vi "Simple SFTP File Download.vi"() -> ()   [LabVIEW 2018]
doc: "Downloads, or receives, a relatively small file from a remote SFTP server. This is similar to the SFTP command line utility when transferring, or copying, a remote file to a local destination. If performance is poor or memory is limited on the local machine, then it could be because the file is relatively large and this implementation is not very efficient for relatively large files."
uses:
  Toolkit/SFTP Attributes/SFTP Attributes.lvclass/SFTP Attributes.ctl
  Toolkit/SSH/SSH.lvclass/SSH.ctl
  Toolkit/SSH/Utility/Read Shared Library.vi
  Toolkit/Session/Support/Create from SSH.vi
  Toolkit/Session/Support/Password Authentication.vi
  Toolkit/SFTP/Support/Create from Session.vi
  Toolkit/SFTP File/Support/Open from SFTP.vi
  Toolkit/SFTP Attributes/Support/Create from SFTP File.vi
  Toolkit/Support/Check Status.vi
  Toolkit/SFTP Attributes/Support/Destroy to SFTP File.vi
  Toolkit/SFTP File/Support/Close to SFTP.vi
  Toolkit/SFTP/Support/Destroy to Session.vi
  Toolkit/Session/Support/Destroy to SSH.vi
  Toolkit/SSH/SSH.lvclass
  Toolkit/Session/Session.lvclass
  Toolkit/SFTP/SFTP.lvclass
  Toolkit/SFTP File/SFTP File.lvclass
  Toolkit/SFTP Attributes/SFTP Attributes.lvclass
panel:
  in  "Remote File":string
  in  "Local File":path
  in  "Remote SFTP Server":string
  in  "Password":string
  in  "Username":string
  # "Overview: Demonstrates transferring, or downloading, a remote file from a SSH server, similar to the SFTP command line utility\nInstructions:\n1. Enter the IP address or host name of the remote SFTP server. This can be a CompactRIO (cRIO) running the National Instruments Linux Real-Time (NI Linux RT) operating system with the Enable Secure Shell Server (sshd) checkbox checked. \n2. Enter a username. If using a cRIO with a default configuration, then the username is \"admin\".\n3. Enter a password for the username. If using a cRIO with a default configuration, then the password is blank (empty).\n4. Enter the path and/or filename of the remote file to download. Typically, this is a POSIX/UNIX file path with a backslash, \"/\", used to separate directories and the default directory is the remote user's home directory, i.e. \"/home/admin\" on a default configured cRIO.\n5. Select a destination on the local computer for the transfer/download from the remote SSH server.\n6. Run this VI."
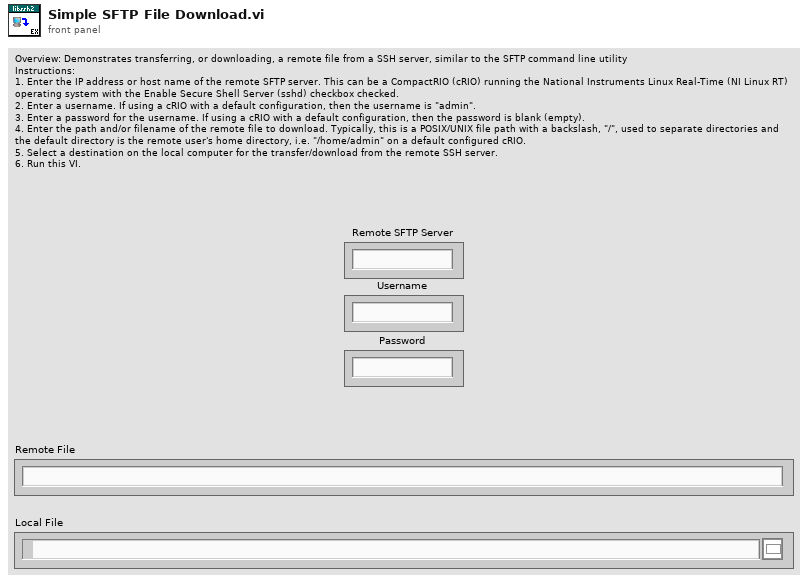
[diagram p1: front panel]
types:
  T1 = enum16{"open", "replace", "create", "open or create", "replace or create", "replace or create with confirmation"}
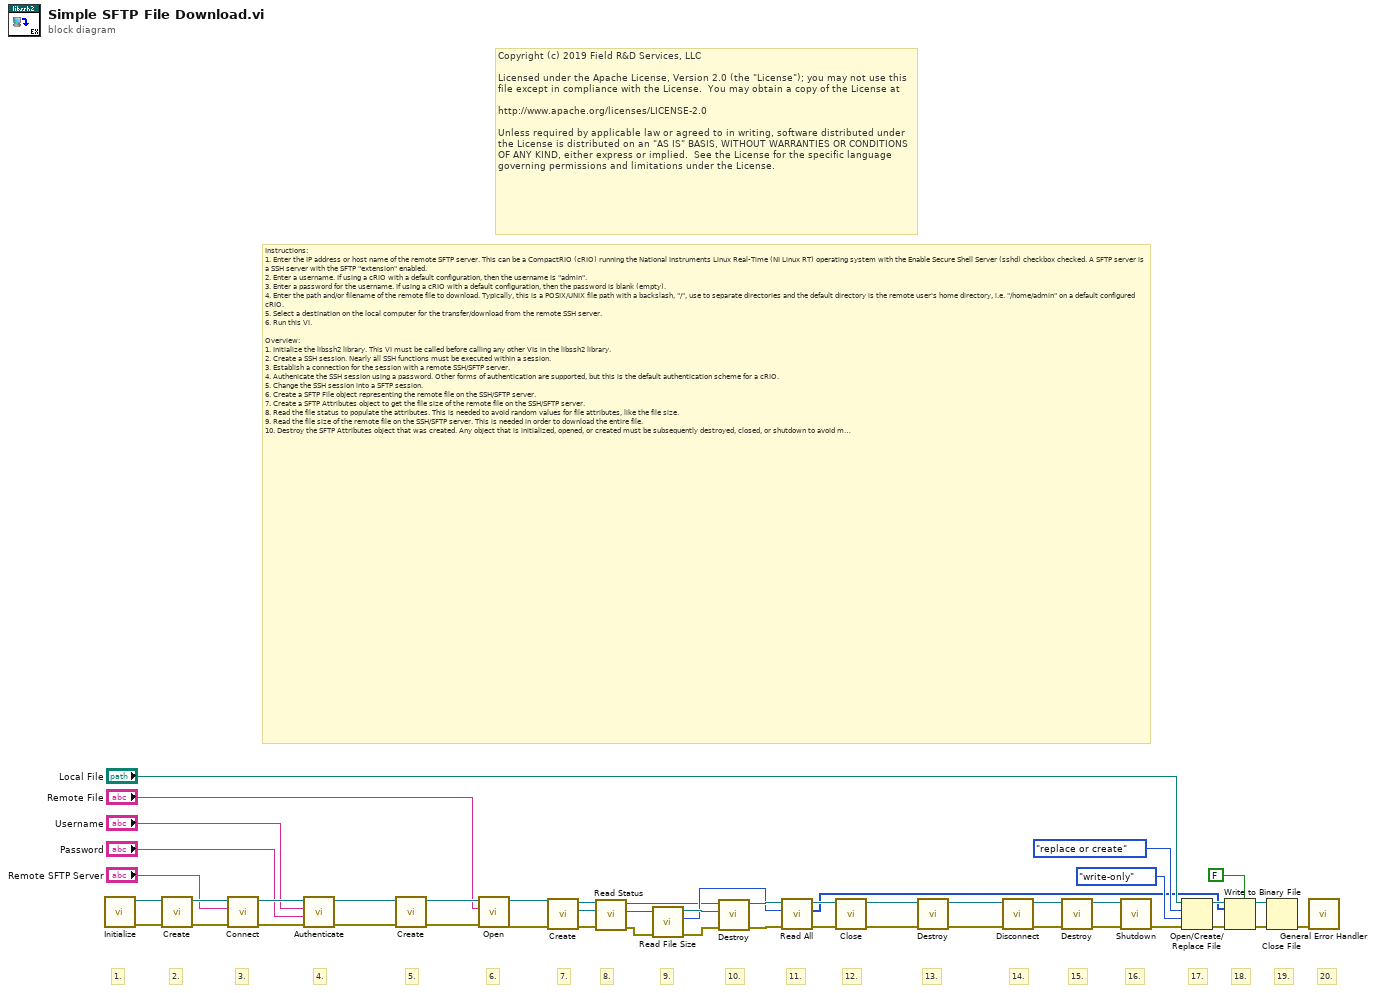
[diagram p0: block diagram]
diagram:
  # "8."
  # "20."
  # "19."
  # "18."
  # "17."
  # "16."
  # "Copyright (c) 2019 Field R&D Services, LLC\n\nLicensed under the Apache License, Version 2.0 (the \"License\"); you may not use this file except in compliance with the License.  You may obtain a copy of the License at\n\nhttp://www.apache.org/licenses/LICENSE-2.0\n\nUnless required by applicable law or agreed to in writing, software distributed under the License is distributed on an \"AS IS\" BASIS, WITHOUT WARRANTIES OR CONDITIONS OF ANY KIND, either express or implied.  See the License for the specific language governing permissions and limitations under the License."
  # "15."
  # "14."
  # "13."
  # "12."
  # "11."
  # "10."
  # "9."
  # "7."
  # "6."
  # "5."
  # "4."
  # "3."
  # "2."
  # "1."
  # "Instructions:\n1. Enter the IP address or host name of the remote SFTP server. This can be a CompactRIO (cRIO) running the National Instruments Linux Real-Time (NI Linux RT) operating system with the Enable Secure Shell Server (sshd) checkbox checked. A SFTP server is a SSH server with the SFTP \"extension\" enabled.\n2. Enter a username. If using a cRIO with a default configuration, then the username is \"admin\".\n3. Enter a password for the username. If using a cRIO with a default configuration, then the password is blank (empty).\n4. Enter the path and/or filename of the remote file to download. Typically, this is a POSIX/UNIX file path with a backslash, \"/\", use to separate directories and the default directory is the remote user's home directory, i.e. \"/home/admin\" on a default configured cRIO.\n5. Select a destination on the local computer for the transfer/download from the remote SSH server.\n6. Run this VI.\n\nOverview:\n1. Initialize the libssh2 library. This VI must be called before calling any other VIs in the libssh2 library.\n2. Create a SSH session. Nearly all SSH functions must be executed within a session.\n3. Establish a connection for the session with a remote SSH/SFTP server.\n4. Authenicate the SSH session using a password. Other forms of authentication are supported, but this is the default authentication scheme for a cRIO. \n5. Change the SSH session into a SFTP session.\n6. Create a SFTP File object representing the remote file on the SSH/SFTP server.\n7. Create a SFTP Attributes object to get the file size of the remote file on the SSH/SFTP server.\n8. Read the file status to populate the attributes. This is needed to avoid random values for file attributes, like the file size.\n9. Read the file size of the remote file on the SSH/SFTP server. This is needed in order to download the entire file.\n10. Destroy the SFTP Attributes object that was created. Any object that is initialized, opened, or created must be subsequently destroyed, closed, or shutdown to avoid memory leaks, undefined behavior, or crashes.\n11. Read all of the bytes from the remote file. This is not the most efficient implementation. A different implementation that reads the remote file in blocks, or chucks, maybe needed if performance is poor or the file is relatively large.\n12. Close the SFTP file on the remote SSH/SFTP server. Any object that is initialized, opened, or created must be subsequently destroyed, closed, or shutdown to avoid memory leaks, undefined behavior, or crashes.\n13. Change the SFTP session back into a SSH session.\n14. Disconnect from the remote SSH server.\n15. Destroy the session to free resources within the libssh2 library.\n16. Shutdown the libssh2 library. This VI must be last VI called for the libssh2 library. No other libssh2 VIs should be called once this VI is executed.\n17. Create or replace (overwrite) a file to write the read contents from the remote file.\n18. Write the data from the remote file.\n19. Close the file. This is not strictly necessary, but it is good practice.\n20. Provide basic error handling.\n19. Provide some error handling and reporting. Libssh2 errors will be in the -8100 range."
  n1 = call "Initialize.vi"() -> ("Error Out"=w37:errorcluster, "SSH"=w36:refnum<class "SSH.lvclass">)  [unwired: 10 in]
  n2 = call-poly "Create.vi"("Error In"=w37, "SSH"=w36) -> ("Error Out"=w47:errorcluster, "Sesssion"=w48:refnum<class "Session.lvclass">)  [unwired: 8 in]
  n3 = call "Connect.vi"("Error In"=w47, "Address"="Remote SFTP Server", "Session In"=w48) -> ("Error Out"=w45:errorcluster, "Sesssion Out"=w46:refnum<class "Session.lvclass">)  [unwired: 7 in]
  n4 = call-poly "Authenticate.vi"("Error In"=w45, "Password"="Password", "Username"="Username", "Session In"=w46) -> ("Error Out"=w25:errorcluster, "Sesssion Out"=w26:refnum<class "Session.lvclass">)  [unwired: 6 in]
  n5 = call-poly "Create.vi"("Error In"=w25, "Session"=w26) -> ("Error Out"=w23:errorcluster, "SFTP"=w24:refnum<class "SFTP.lvclass">)  [unwired: 8 in]
  n6 = call-poly "Open.vi"("Error In"=w23, "Remote Path"="Remote File", "SFTP"=w24) -> ("Error Out"=w20:errorcluster, "SFTP File"=w21:refnum<class "SFTP File.lvclass">)  [unwired: 7 in]
  n7 = call-poly "Create.vi"("Error In"=w20, "SFTP File In"=w21) -> ("Error Out"=w2:errorcluster, "SFTP Attributes"=w3:refnum<class "SFTP Attributes.lvclass">, "SFTP File Out"=w6:refnum<class "SFTP File.lvclass">)  [unwired: 7 in]
  n8 = call "Read Status.vi"("Error In"=w2, "Attributes In"=w3, "SFTP File In"=w6) -> ("Error Out"=w1:errorcluster, "Attributes Out"=w4:refnum<class "SFTP Attributes.lvclass">, "SFTP File Out"=w5:refnum<class "SFTP File.lvclass">)  [unwired: 6 in]
  n9 = call "Read File Size.vi"("Error In"=w1, "SFTP Attributes In"=w4) -> ("Error Out"=w14:errorcluster, "File Size"=w8:u64, "SFTP Attributes Out"=w15:refnum<class "SFTP Attributes.lvclass">)  [unwired: 7 in]
  n10 = call-poly "Destroy.vi"("Error In"=w14, "SFTP Attributes"=w15, "SFTP File In"=w5) -> ("Error Out"=w12:errorcluster, "SFTP File Out"=w13:refnum<class "SFTP File.lvclass">)  [unwired: 7 in]
  n11 = call "Read All.vi"("Error In"=w12, "Max Read Size"=w8, "SFTP File In"=w13) -> ("Error Out"=w10:errorcluster, "Data"=w9:u8[], "SFTP File Out"=w11:refnum<class "SFTP File.lvclass">)  [unwired: 6 in]
  n12 = call-poly "Close.vi"("Error In"=w10, "SFTP File"=w11) -> ("Error Out"=w18:errorcluster, "SFTP"=w19:refnum<class "SFTP.lvclass">)  [unwired: 7 in, 1 out]
  n13 = call-poly "Destroy.vi"("Error In"=w18, "SFTP"=w19) -> ("Error Out"=w16:errorcluster, "Session"=w17:refnum<class "Session.lvclass">)  [unwired: 8 in]
  n14 = call "Disconnect.vi"("Error In"=w16, "Session In"=w17) -> ("Error Out"=w40:errorcluster, "Sesssion Out"=w41:refnum<class "Session.lvclass">)  [unwired: 8 in]
  n15 = call-poly "Destroy.vi"("Error In"=w40, "Session"=w41) -> ("Error Out"=w38:errorcluster, "SSH"=w39:refnum<class "SSH.lvclass">)  [unwired: 8 in]
  n16 = call "Shutdown.vi"("Error In"=w38, "SSH"=w39) -> ("Error Out"=w35:errorcluster)  [unwired: 9 in]
  n17 = Open/Create/Replace File(file path (use dialog)="Local File", error in=w35, operation (0:open)=T1."replace or create", access (0:read/write)=enum16{"read/write", "read-only", "write-only"}."write-only") -> (refnum out=w31:refnum<file>, error out=w30:errorcluster)  [unwired: 2 in, 1 out]
  n18 = Write to Binary File(file (use dialog)=w31, data=w9, error in=w30, 5:FALSE ("prepend array or string size? (T)")) -> (refnum out=w29:refnum<file>, error out=w28:errorcluster)  [unwired: 2 in, 1 out]
  n19 = Close File(refnum=w29, error in=w28) -> (error out=w27:errorcluster)  [unwired: 1 out]
  n20 = call <vilib>:"General Error Handler.vi"("error in (no error)"=w27) -> ()  [unwired: 10 in, 5 out]
